vi "test_queue2.vi"() -> ()   [LabVIEW 2012]
doc: "Use this template to build a producer/consumer design pattern. Use this template when you need to execute a process, such as data analysis, when a data source, such as a triggered acquisition, produces data at an uneven rate and you need to execute the process when the data becomes available."
panel:
  out "Tableau":string[][](array[string])
  out "1-D array":string[](array[string])
  out "Cluster":T1
  in  "stop":bool
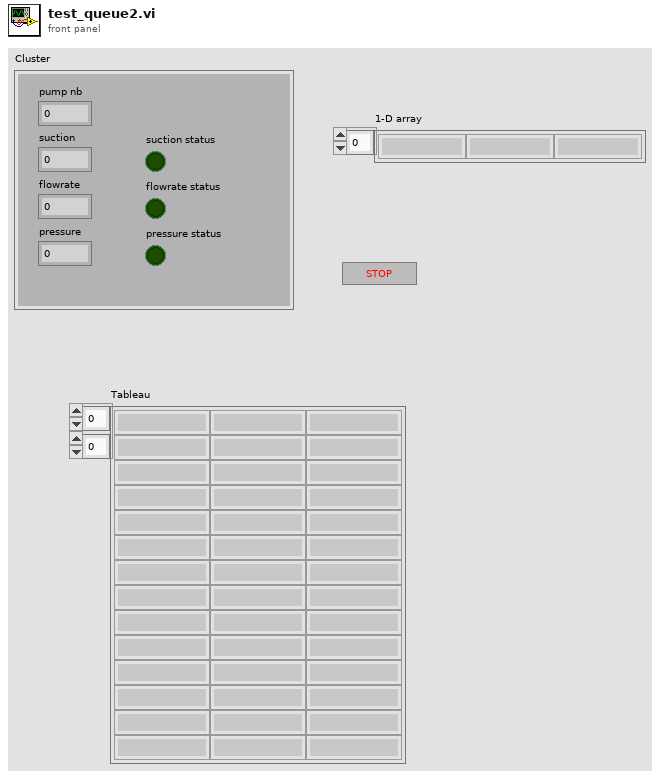
[diagram p1: front panel]
types:
  T1 = cluster{"pump nb":dbl, "suction":dbl, "suction status":bool, "flowrate":dbl, "flowrate status":bool, "pressure":dbl, "pressure status":bool}
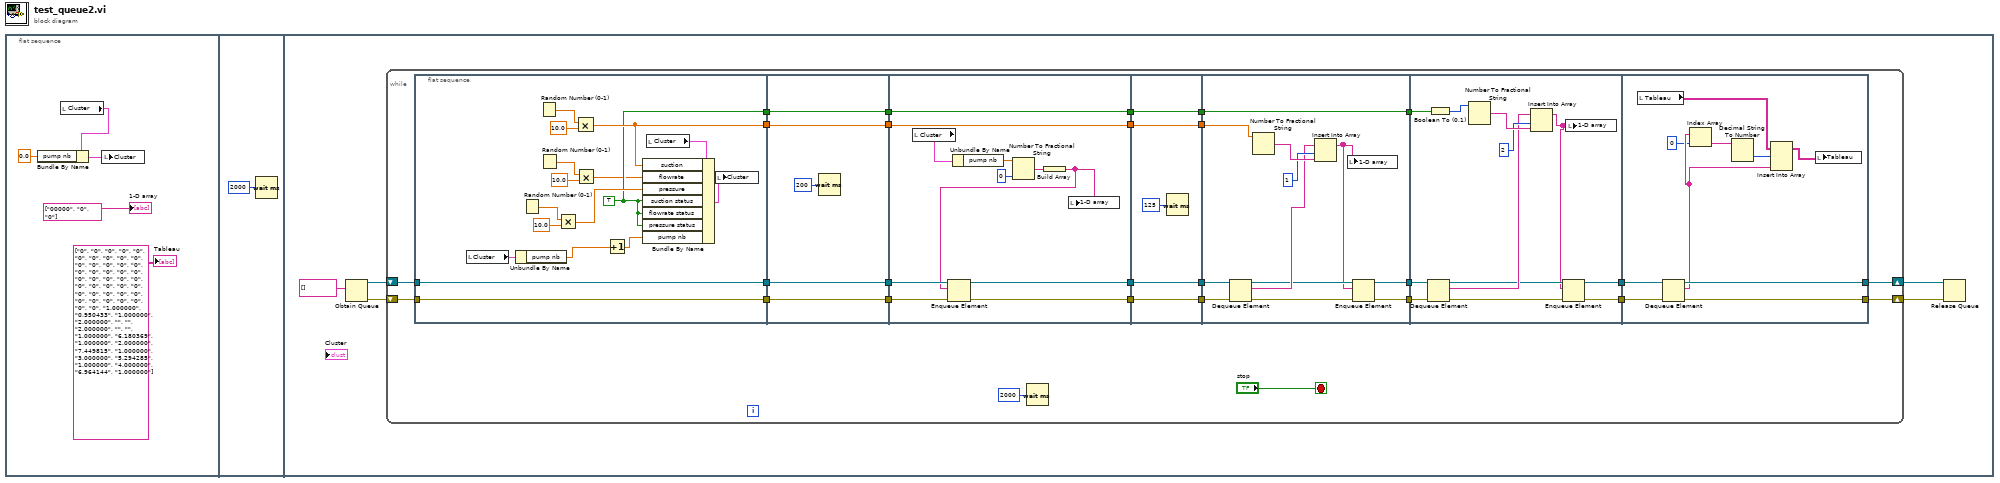
[diagram p0: block diagram]
diagram:
  n1 = flat-sequence {
    frame #0 {
      n2 = local read "Cluster"() -> (w4:T1)
      n3 = Bundle By Name(cluster=w4, "pump nb"=0.0) -> (w3:T1)
      n4 = local write "Cluster"(w3) -> ()
      "1-D array" <- string[] ["00000", "0", "0"] ("1-D array")
      "Tableau" <- string[][] [["0", "0", "0"], ["0", "0", "0"], ["0", "0", "0"], ["0", "0", "0"], ["0", "0", "0"], ["0", "0", "0"], ["0", "0", "0"], ["0", "0", "0"], ["0", "0", "0"], ["0", "0", "0"], ["0", "0", "0"], ["0", "0", "0"], ["0", "0", "0"], ["0", "0", "0"], ["1.000000", "0.950433", "1.000000"], ["2.000000", "", ""], ["2.000000", "", ""], ["1.000000", "6.180369", "1.000000"], ["2.000000", "7.449815", "1.000000"], ["3.000000", "5.294285", "1.000000"], ["4.000000", "6.964144", "1.000000"]] ("Tableau")
    }
    frame #1 {
      n5 = Wait (ms)(milliseconds to wait=u32 2000) -> ()  [unwired: 1 out]
    }
    frame #2 {
      n6 = Obtain Queue(element data type=string[] []) -> (queue out=w11:refnum<queue>, error out=w10:errorcluster)  [unwired: 4 in, 1 out]
      n7 = while {
        shift-right: [w35] -> w8
        shift-left: w10 -> [w37]
        shift-right: [w36] -> w9
        shift-left: w11 -> [w38]
        stop <- "stop" stop-if-true
        n8 = flat-sequence {
          tunnel: w37 -> [w54]
          tunnel: w38 -> [w55]
          tunnel: [w55] -> w31
          tunnel: [w54] -> w30
          tunnel: [w41] -> w23
          tunnel: [w40] -> w14
          tunnel: [w60] -> w33
          tunnel: [w59] -> w32
          tunnel: w31 -> [w60]
          tunnel: w30 -> [w59]
          tunnel: [w57] -> w24
          tunnel: w23 -> [w57]
          tunnel: [w56] -> w15
          tunnel: w14 -> [w56]
          tunnel: [w69] -> w22
          tunnel: [w68] -> w20
          tunnel: w33 -> [w71]
          tunnel: w32 -> [w70]
          tunnel: [w63] -> w18
          tunnel: w24 -> [w63]
          tunnel: [w62] -> w16
          tunnel: w15 -> [w62]
          tunnel: w22 -> [w76]
          tunnel: [w76] -> w21
          tunnel: w20 -> [w75]
          tunnel: [w75] -> w19
          tunnel: w18 -> [w74]
          tunnel: [w74] -> w17
          tunnel: w16 -> [w72]
          tunnel: [w72] -> w13
          tunnel: w21 -> [w88]
          tunnel: w19 -> [w87]
          tunnel: [w80] -> w28
          tunnel: [w78] -> w26
          tunnel: w17 -> [w86]
          tunnel: w13 -> [w83]
          tunnel: [w83] -> w12
          tunnel: w28 -> [w100]
          tunnel: [w91] -> w27
          tunnel: w26 -> [w99]
          tunnel: [w90] -> w25
          tunnel: w12 -> [w95]
          tunnel: [w105] -> w35
          tunnel: [w107] -> w36
          tunnel: w27 -> [w108]
          tunnel: w25 -> [w106]
          frame #0 {
            w40 = TRUE ("suction status")
            n9 = local read "Cluster"() -> (w43:T1)
            n10 = Unbundle By Name(w43) -> ("pump nb"=w42:dbl)
            n11 = Random Number (0-1)() -> (number: 0 to 1=w51:dbl)
            n12 = Random Number (0-1)() -> (number: 0 to 1=w45:dbl)
            n13 = Random Number (0-1)() -> (number: 0 to 1=w49:dbl)
            n14 = Multiply(x=w51, y=10.0) -> (x*y=w53:dbl)
            n15 = Multiply(x=w45, y=10.0) -> (x*y=w41:dbl)
            n16 = Multiply(x=w49, y=10.0) -> (x*y=w39:dbl)
            n17 = Increment(x=w42) -> (x+1=w44:dbl)
            n18 = local read "Cluster"() -> (w47:T1)
            n19 = Bundle By Name(cluster=w47, "suction"=w41, "flowrate"=w39, "pressure"=w53, "suction status"=w40, "flowrate status"=w40, "pressure status"=w40, "pump nb"=w44) -> (w48:T1)
            n20 = local write "Cluster"(w48) -> ()
          }
          frame #1 {
            n21 = Wait (ms)(milliseconds to wait=u32 200) -> ()  [unwired: 1 out]
          }
          frame #2 {
            n22 = local read "Cluster"() -> (w67:T1)
            n23 = Unbundle By Name(w67) -> ("pump nb"=w64:dbl)
            n24 = Number To Fractional String(number=w64, precision (6)=i16 0) -> (F-format string=w66:string)  [unwired: 2 in]
            n25 = Build Array(w66) -> (w65:string[])
            n26 = Enqueue Element(queue=w71, element=w65, error in (no error)=w70) -> (queue out=w69:refnum<queue>, error out=w68:errorcluster)  [unwired: 1 in, 1 out]
            n27 = local write "1-D array"(w65) -> ()
          }
          frame #3 {
            n28 = Wait (ms)(milliseconds to wait=u32 125) -> ()  [unwired: 1 out]
          }
          frame #4 {
            n29 = Dequeue Element(queue=w88, error in (no error)=w87) -> (queue out=w81:refnum<queue>, element=w82:string[], error out=w79:errorcluster)  [unwired: 1 in, 1 out]
            n30 = Number To Fractional String(number=w86) -> (F-format string=w85:string)  [unwired: 3 in]
            n31 = Insert Into Array(array=w82, index=1, new element=w85) -> (w77:string[])
            n32 = local write "1-D array"(w77) -> ()
            n33 = Enqueue Element(queue=w81, element=w77, error in (no error)=w79) -> (queue out=w80:refnum<queue>, error out=w78:errorcluster)  [unwired: 1 in, 1 out]
          }
          frame #5 {
            n34 = Dequeue Element(queue=w100, error in (no error)=w99) -> (queue out=w92:refnum<queue>, element=w96:string[], error out=w93:errorcluster)  [unwired: 1 in, 1 out]
            n35 = Boolean To (0,1)(Boolean=w95) -> (0, 1=w94:i16)
            n36 = Number To Fractional String(number=w94) -> (F-format string=w98:string)  [unwired: 3 in]
            n37 = Insert Into Array(array=w96, index=2, new element=w98) -> (w89:string[])
            n38 = Enqueue Element(queue=w92, element=w89, error in (no error)=w93) -> (queue out=w91:refnum<queue>, error out=w90:errorcluster)  [unwired: 1 in, 1 out]
            n39 = local write "1-D array"(w89) -> ()
          }
          frame #6 {
            n40 = local read "Tableau"() -> (w110:string[][])
            n41 = Dequeue Element(queue=w108, error in (no error)=w106) -> (queue out=w107:refnum<queue>, element=w104:string[], error out=w105:errorcluster)  [unwired: 1 in, 1 out]
            n42 = Index Array(array=w104, index=0) -> (element=w101:string)
            n43 = Decimal String To Number(string=w101) -> (number=w102:i32)  [unwired: 2 in, 1 out]
            n44 = Insert Into Array(array=w110, index (row)=w102, new element=w104) -> (w109:string[][])  [unwired: 1 in]
            n45 = local write "Tableau"(w109) -> ()
          }
        }
        n46 = Wait (ms)(milliseconds to wait=u32 2000) -> ()  [unwired: 1 out]
      }
      n47 = Release Queue(queue=w9, error in (no error)=w8) -> ()  [unwired: 1 in, 3 out]
    }
  }
